vi "Get Short.vi"(8 "error in (no error)":errorcluster, 11 "Uint64 in":refnum<class "Uint64.lvclass">) -> (0 "error out":errorcluster, 2 "I16 out":i16, 3 "Uint64 out":refnum<class "Uint64.lvclass">)   [LabVIEW 2015, in "MDSplus.lvlib" / "Uint64.lvclass"]
uses:
  <vilib>/MDSplus/Classes/Data_Class/Scalar_Class/Uint64_Class/Uint64.lvclass
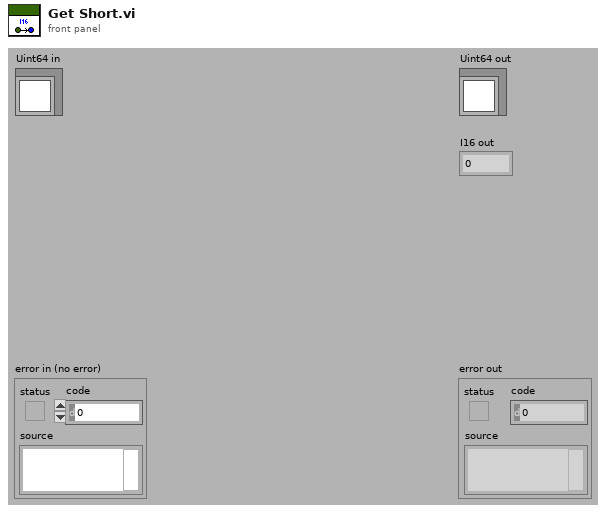
[diagram p1: front panel]
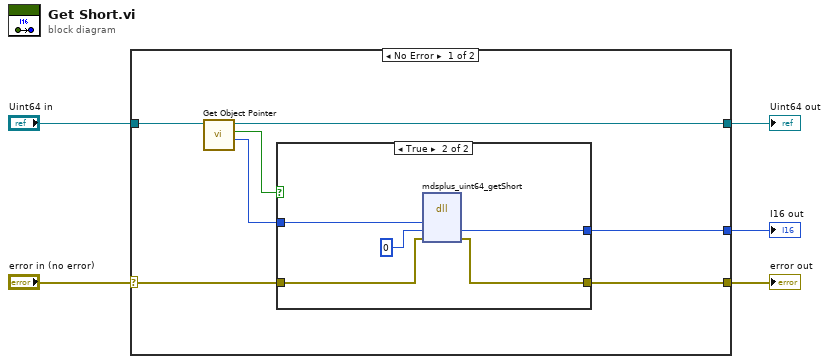
[diagram p0: block diagram]
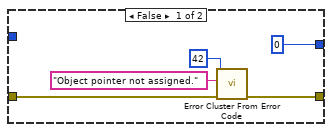
[diagram p2: hidden frame]
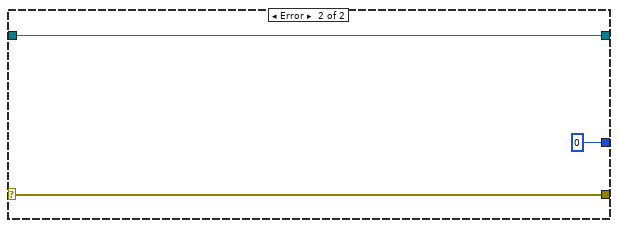
[diagram p3: hidden frame]
diagram:
  n1 = case shown="No Error" "error in (no error)" {
    selector: "error in (no error)" -> [w8 w25]
    tunnel: [w7 w25] -> w4
    tunnel: [w6 w24] -> w2
    tunnel: "Uint64 in" -> [w12 w24]
    tunnel: [w11 i16 0 ("floatOut")] -> w1
    frame No Error {
      n2 = call-dynamic "Get Object Pointer.vi"("Data in"=w12) -> ("Object Pointer"=w9:i64, "Assigned object pointer?"=w10:bool, "Data out"=w6:refnum<class "Uint64.lvclass">)  [unwired: 8 in]
      n3 = case shown="True" w10 {
        tunnel: [i16 0 ("floatOut") w21] -> w11
        tunnel: w9 -> [_ w20]
        tunnel: w8 -> [w14 w19]
        tunnel: [w13 w18] -> w7
        frame False {
          n4 = call <vilib>:"Error Cluster From Error Code.vi"("error in (no error)"=w14, "error message (\"\")"="Object pointer not assigned." ("error message (\"\")"), "error code (0)"=42) -> ("error out"=w13:errorcluster)  [unwired: 6 in]
        }
        frame True {
          n5 = dll-call lib="MDSobjectsLVShr" fn="mdsplus_uint64_getShort"("lvUint64Ptr"=w20, "shortOut"=i16 0 ("floatOut"), "error"=w19) -> ("shortOut"=w21:i16, "error"=w18:errorcluster)  [unwired: 5 in, 2 out]
        }
      }
    }
    frame Error {
    }
  }
  "error out" <- w4
  "Uint64 out" <- w2
  "I16 out" <- w1
